vi "Input impedance.vi"() -> ()   [LabVIEW 2017]
panel:
  out "ph1-ph2":dbl
  out "A2":dbl
  out "A1":dbl
  out "ph1-ph2 graph":cluster{"Y":dbl[], "Y":dbl[]}[](graph)
  out "A2 graph":cluster{"Y":dbl[], "Y":dbl[]}[](graph)
  out "A1 graph":cluster{"Y":dbl[], "Y":dbl[]}[](graph)
  out "Im Z 2":dbl=nan
  out "Re Z 2":dbl=nan
  out "Im (Z)":cluster{"Y":dbl[], "Y":dbl[]}[](graph)
  out "Re (Z)":cluster{"Y":dbl[], "Y":dbl[]}[](graph)
  out "Arg (Z)":cluster{"Y":dbl[], "Y":dbl[]}[](graph)
  out "Abs (Z)":cluster{"Y":dbl[], "Y":dbl[]}[](graph)
  out "Abs Z 2":dbl=nan
  out "Arg Z 2":dbl=nan
  in  "Resistance (Ohm)":dbl=162.0
  in  "Commentary":string
  in  "horiz range factor":dbl=0.3
  in  "vert range factor":dbl=1.2
  out "frequency":dbl=20010000.0
  out "datafile":refnum<file>
  in  "Min f":dbl=10000.0
  in  "Channel 2 preset commands":string=":channel2:bwlimit 0\n:channel2:coupling AC\n:channel2:display 1\n:channel2:invert 0\n:channel2:offset 0"
  in  "Channel 1 preset commands":string=":channel1:bwlimit 0\n:channel1:coupling AC\n:channel1:display 1\n:channel1:invert 0\n:channel1:offset 0\n"
  in  "Ampl":dbl=9.0
  in  "Source preset commands":string=":WGEN:OUTPut 1\n:WGEN:VOLTage:OFFSet 1e-6\n:WGEN:OUTPut:LOAD FIFTy\n:wgen:function sinusoid\n:WGEN:OUTPut:POLarity 0\n"
  in  "Delta f":dbl=10000.0
  in  "Max f":dbl=20000000.0
  in  "Timeout Value (ms)":u32=5000
  in  "VISA resource name":refnum<visa-resource-name>="USB0::0x2A8D::0x1797::CN58056487::INSTR"
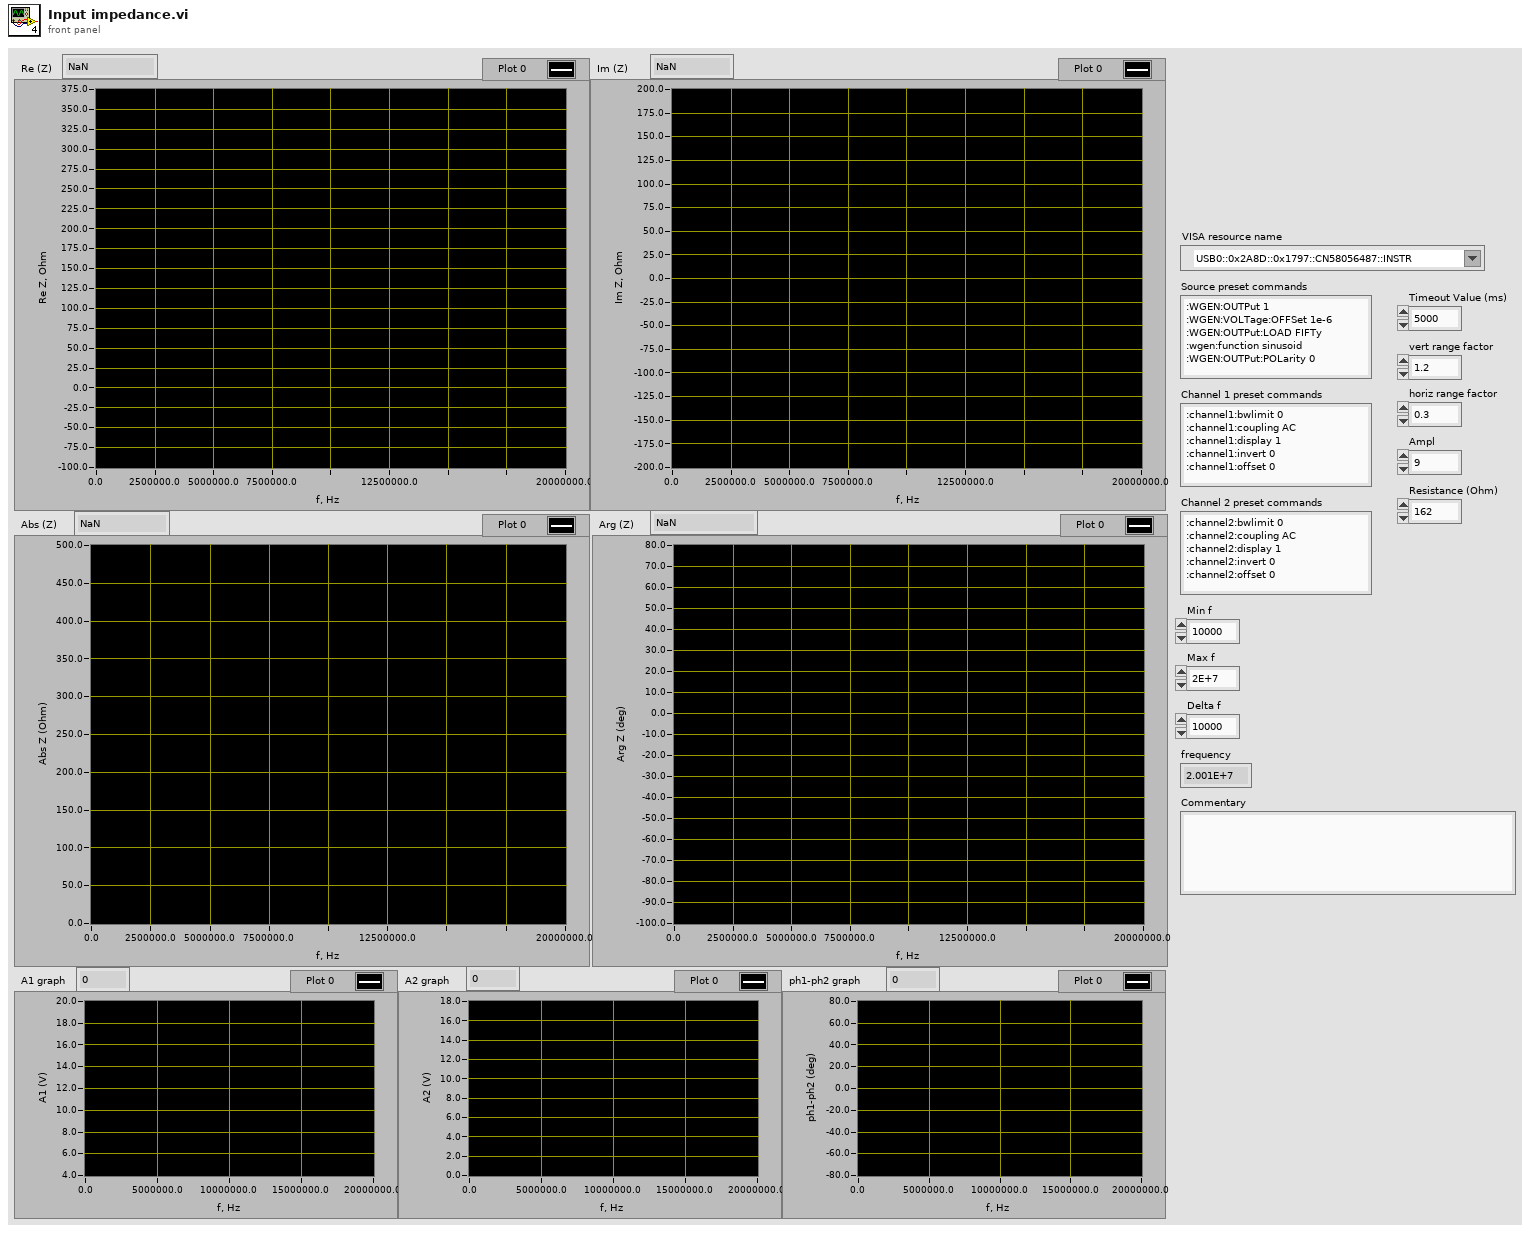
[diagram p1: front panel]
types:
  T1 = enum16{"open", "replace", "create", "open or create", "replace or create", "replace or create with confirmation"}
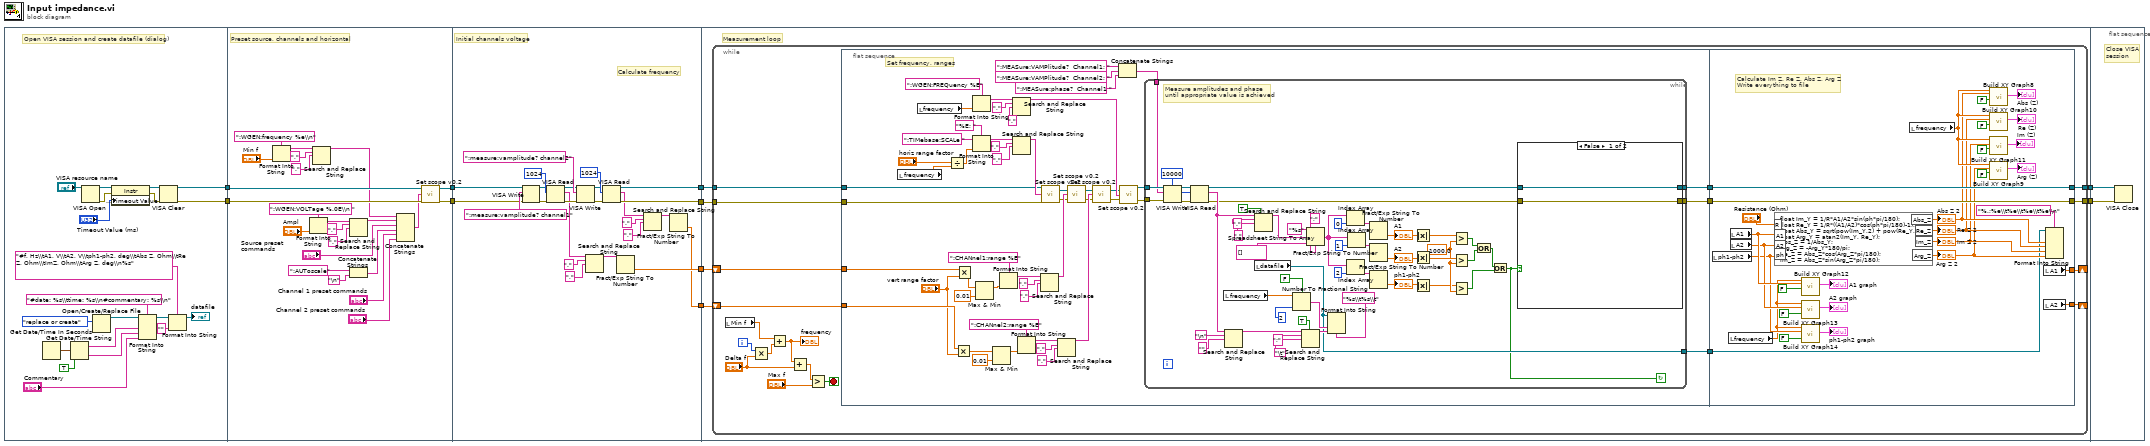
[diagram p0: block diagram]
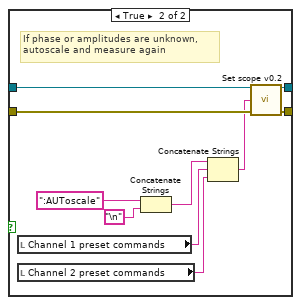
[diagram p2: hidden frame]
diagram:
  n1 = flat-sequence {
    tunnel: [w23] -> w10
    tunnel: [w24] -> w9
    tunnel: [w53] -> w8
    tunnel: [w52] -> w7
    tunnel: w9 -> [w50]
    tunnel: w10 -> [w51]
    tunnel: w8 -> [w67]
    tunnel: w7 -> [w66]
    tunnel: [w59] -> w6
    tunnel: [w54] -> w5
    tunnel: [w65] -> w4
    tunnel: [w64] -> w3
    tunnel: w6 -> [w83]
    tunnel: w5 -> [w82]
    tunnel: w4 -> [w81]
    tunnel: w3 -> [w80]
    tunnel: [w79] -> w2
    tunnel: [w78] -> w1
    tunnel: w2 -> [w247]
    tunnel: w1 -> [w246]
    frame #0 {
      # "Open VISA session and create datafile (dialog)"
      n2 = Get Date/Time In Seconds() -> (seconds since 1Jan1904=w20:timestamp)
      n3 = Get Date/Time String(seconds (now)=w20, want seconds? (F)=TRUE) -> (date string=w17:string, time string=w16:string)  [unwired: 1 in]
      n4 = VISA Open(VISA resource name="VISA resource name") -> (VISA resource name=w28:refnum<visa-resource-name>, error out=w29:errorcluster)  [unwired: 4 in]
      n5 = Open/Create/Replace File(operation (0:open)=T1."replace or create") -> (refnum out=w21:refnum<file>)  [unwired: 5 in, 2 out]
      n6 = property class="Instr"(reference=w28, error in=w29, "General Settings:Timeout Value"="Timeout Value (ms)") -> (reference out=w26:refnum<visa-resource-name>, error out=w25:errorcluster)
      n7 = Format Into String(format string="#date: %s\\ttime: %s\\n#commentary: %s\\n", initial string=w21, w17, w16, "Commentary") -> (resulting string=w13:refnum<file>)  [unwired: 1 in, 1 out]
      n8 = VISA Clear(VISA resource name=w26, error in (no error)=w25) -> (VISA resource name out=w23:refnum<visa-resource-name>, error out=w24:errorcluster)
      n9 = Format Into String(format string="#f, Hz\\tA1, V\\tA2, V\\tph1-ph2, deg\\tAbs Z, Ohm\\tRe Z, Ohm\\tImZ, Ohm\\tArg Z, deg\\n%s", initial string=w13, "" ("input 1")) -> (resulting string=→"datafile":refnum<file>)  [unwired: 1 in, 1 out]
    }
    frame #1 {
      # "Preset source, channels and horizontal"
      n10 = Format Into String(format string=":WGEN:frequency %e\\n", "Min f") -> (resulting string=w39:string)  [unwired: 2 in, 1 out]
      n11 = Format Into String(format string=":WGEN:VOLTage %.0E\\n ", "Ampl") -> (resulting string=w45:string)  [unwired: 2 in, 1 out]
      n12 = Search and Replace String(input string=w39, search string="," ("replace string (\"\")"), replace string="." ("replace string (\"\")")) -> (result string=w36:string)  [unwired: 5 in, 3 out]
      n13 = Search and Replace String(input string=w45, search string="," ("replace string (\"\")"), replace string="." ("replace string (\"\")")) -> (result string=w43:string)  [unwired: 5 in, 3 out]
      n14 = Concatenate Strings(":AUToscale" ("write buffer"), "\n") -> (w33:string)
      n15 = Concatenate Strings(w36, w43, "Source preset commands", w33, "Channel 1 preset commands", "Channel 2 preset commands") -> (w44:string)
      n16 = call "Set scope v0.2.vi"("error in (no error)"=w50, "input commands"=w44, "VISA resource name in"=w51) -> ("error out"=w52:errorcluster, "VISA resource name out"=w53:refnum<visa-resource-name>)
    }
    frame #2 {
      # "Calculate frequency"
      # "Initial channels voltage"
      n17 = VISA Write(VISA resource name=w67, write buffer=":measure:vamplitude? channel1", error in (no error)=w66) -> (VISA resource name out=w71:refnum<visa-resource-name>, error out=w70:errorcluster)  [unwired: 1 out]
      n18 = VISA Read(VISA resource name=w71, byte count=u32 1024, error in (no error)=w70) -> (VISA resource name out=w72:refnum<visa-resource-name>, read buffer=w61:string, error out=w73:errorcluster)  [unwired: 1 out]
      n19 = VISA Write(VISA resource name=w72, write buffer=":measure:vamplitude? channel2", error in (no error)=w73) -> (VISA resource name out=w69:refnum<visa-resource-name>, error out=w68:errorcluster)  [unwired: 1 out]
      n20 = Search and Replace String(input string=w61, search string="." ("replace string (\"\")"), replace string="," ("replace string (\"\")")) -> (result string=w60:string)  [unwired: 5 in, 3 out]
      n21 = VISA Read(VISA resource name=w69, byte count=u32 1024, error in (no error)=w68) -> (VISA resource name out=w65:refnum<visa-resource-name>, read buffer=w55:string, error out=w64:errorcluster)  [unwired: 1 out]
      n22 = Fract/Exp String To Number(string=w60) -> (number=w59:dbl)  [unwired: 3 in, 1 out]
      n23 = Search and Replace String(input string=w55, search string="." ("replace string (\"\")"), replace string="," ("replace string (\"\")")) -> (result string=w56:string)  [unwired: 5 in, 3 out]
      n24 = Fract/Exp String To Number(string=w56) -> (number=w54:dbl)  [unwired: 3 in, 1 out]
    }
    frame #3 {
      # "Measurement loop"
      n25 = while {
        shift-right: [w92] -> _
        shift-left: w83 -> [w102]
        shift-right: [w93] -> _
        shift-left: w82 -> [w101]
        tunnel: w81 -> [w100]
        tunnel: w80 -> [w99]
        tunnel: [w98] -> w79
        tunnel: [w97] -> w78
        i -> [w87]
        stop <- w89 stop-if-true
        n26 = local read "Min f"() -> (w91:dbl)
        n27 = Multiply(x=w87, y="Delta f") -> (x*y=w90:dbl)
        n28 = Add(x=w91, y=w90) -> (x+y=w88:dbl)
        "frequency" <- w88
        n29 = Add(x=w88, y="Delta f") -> (x+y=w85:dbl)
        n30 = Greater?(x=w85, y="Max f") -> (0:w89:bool)
        n31 = flat-sequence {
          tunnel: [w105] -> w95
          tunnel: [w103] -> w96
          tunnel: [w104] -> w94
          tunnel: w99 -> [w122]
          tunnel: w100 -> [w123]
          tunnel: w101 -> [w120]
          tunnel: w102 -> [w121]
          tunnel: [w244] -> w97
          tunnel: [w245] -> w98
          tunnel: w95 -> [w245]
          tunnel: w96 -> [w222]
          tunnel: w94 -> [w244]
          tunnel: [w217] -> w93
          tunnel: [w216] -> w92
          frame #0 {
            # "Set frequency, ranges"
            n32 = local read "frequency"() -> (w128:dbl)
            n33 = local read "frequency"() -> (w129:dbl)
            n34 = Divide(x="horiz range factor", y=w128) -> (x/y=w148:dbl)
            n35 = Multiply(x=w120, y="vert range factor") -> (x*y=w133:dbl)
            n36 = Multiply(x=w121, y="vert range factor") -> (x*y=w139:dbl)
            n37 = Format Into String(format string="%E; ", initial string=":TIMebase:SCALe " ("write buffer"), w148) -> (resulting string=w149:string)  [unwired: 1 in, 1 out]
            n38 = Format Into String(format string=":WGEN:FREQuency %E", w129) -> (resulting string=w152:string)  [unwired: 2 in, 1 out]
            n39 = Max & Min(x=w139, y=0.01) -> (max(x,y)=w137:dbl)  [unwired: 1 out]
            n40 = Max & Min(x=w133, y=0.01) -> (max(x,y)=w131:dbl)  [unwired: 1 out]
            n41 = Format Into String(format string=":CHANnel1:range %E", w137) -> (resulting string=w143:string)  [unwired: 2 in, 1 out]
            n42 = Search and Replace String(input string=w152, search string="," ("replace string (\"\")"), replace string="." ("replace string (\"\")")) -> (result string=w115:string)  [unwired: 5 in, 3 out]
            n43 = Search and Replace String(input string=w149, search string="," ("replace string (\"\")"), replace string="." ("replace string (\"\")")) -> (result string=w127:string)  [unwired: 5 in, 3 out]
            n44 = Format Into String(format string=":CHANnel2:range %E", w131) -> (resulting string=w136:string)  [unwired: 2 in, 1 out]
            n45 = Search and Replace String(input string=w143, search string="," ("replace string (\"\")"), replace string="." ("replace string (\"\")")) -> (result string=w126:string)  [unwired: 5 in, 3 out]
            n46 = call "Set scope v0.2.vi"("error in (no error)"=w122, "input commands"=w127, "VISA resource name in"=w123) -> ("error out"=w125:errorcluster, "VISA resource name out"=w124:refnum<visa-resource-name>)
            n47 = Search and Replace String(input string=w136, search string="," ("replace string (\"\")"), replace string="." ("replace string (\"\")")) -> (result string=w118:string)  [unwired: 5 in, 3 out]
            n48 = call "Set scope v0.2.vi"("error in (no error)"=w125, "input commands"=w126, "VISA resource name in"=w124) -> ("error out"=w117:errorcluster, "VISA resource name out"=w116:refnum<visa-resource-name>)
            n49 = call "Set scope v0.2.vi"("error in (no error)"=w117, "input commands"=w118, "VISA resource name in"=w116) -> ("error out"=w113:errorcluster, "VISA resource name out"=w114:refnum<visa-resource-name>)
            n50 = Concatenate Strings(":MEASure:VAMPlitude?  Channel1; " ("write buffer"), ":MEASure:VAMPlitude?  Channel2; " ("write buffer"), ":MEASure:phase?  Channel1 " ("write buffer")) -> (w106:string)
            n51 = call "Set scope v0.2.vi"("error in (no error)"=w113, "input commands"=w115, "VISA resource name in"=w114) -> ("error out"=w110:errorcluster, "VISA resource name out"=w111:refnum<visa-resource-name>)
            n52 = while {
              tunnel: w111 -> [w165]
              tunnel: w110 -> [w164]
              tunnel: w106 -> [w163]
              tunnel: [w162] -> w105
              tunnel: [w161] -> w104
              tunnel: [w160] -> w103
              stop <- w154 continue-if-true
              w158 = 1000.0 ("y")
              # "Measure amplitudes and phase\nuntil appropriate value is achieved"
              n53 = VISA Write(VISA resource name=w165, write buffer=w163, error in (no error)=w164) -> (VISA resource name out=w203:refnum<visa-resource-name>, error out=w202:errorcluster)  [unwired: 1 out]
              n54 = VISA Read(VISA resource name=w203, byte count=u32 10000, error in (no error)=w202) -> (VISA resource name out=w187:refnum<visa-resource-name>, read buffer=w193:string, error out=w186:errorcluster)  [unwired: 1 out]
              n55 = local read "frequency"() -> (w194:dbl)
              n56 = Search and Replace String(input string=w193, search string="\n", replace string="" ("replace string (\"\")")) -> (result string=w192:string)  [unwired: 5 in, 3 out]
              n57 = Search and Replace String(replace all?=TRUE ("replace all? (F)"), input string=w193, search string="." ("replace string (\"\")"), replace string="," ("replace string (\"\")")) -> (result string=w201:string)  [unwired: 4 in, 3 out]
              n58 = local read "datafile"() -> (w160:refnum<file>)
              n59 = Number To Fractional String(use system decimal point (T)=FALSE, number=w194, precision (6)=i16 2) -> (F-format string=w197:string)  [unwired: 1 in]
              n60 = Search and Replace String(replace all?=TRUE ("replace all? (F)"), input string=w192, search string=";", replace string="\t") -> (result string=w198:string)  [unwired: 4 in, 3 out]
              n61 = Spreadsheet String To Array(delimiter (Tab)=";", format string="%s", spreadsheet string=w201, array type (2D Dbl)=string[] [] ("initialized array")) -> (array=w196:string[])
              n62 = Format Into String(format string="%s\\t%s\\t", initial string=w160, w197, w198) -> ()  [unwired: 1 in, 2 out]
              n63 = Index Array(array=w196, index=0) -> (element=w200:string)
              n64 = Index Array(array=w196, index=2) -> (element=w195:string)
              n65 = Index Array(array=w196, index=1) -> (element=w199:string)
              n66 = Fract/Exp String To Number(string=w200) -> (number=w191:dbl)  [unwired: 3 in, 1 out]
              "A1" <- w191
              n67 = Fract/Exp String To Number(string=w199) -> (number=w190:dbl)  [unwired: 3 in, 1 out]
              "A2" <- w190
              n68 = Fract/Exp String To Number(string=w195) -> (number=w159:dbl)  [unwired: 3 in, 1 out]
              "ph1-ph2" <- w159
              n69 = Absolute Value(x=w191) -> (abs(x)=w189:dbl)
              n70 = Absolute Value(x=w190) -> (abs(x)=w188:dbl)
              n71 = Absolute Value(x=w159) -> (abs(x)=w157:dbl)
              n72 = Greater?(x=w189, y=w158) -> (0:w185:bool)
              n73 = Greater?(x=w188, y=w158) -> (0:w184:bool)
              n74 = Greater?(x=w157, y=w158) -> (0:w156:bool)
              n75 = Or(x=w185, y=w184) -> (x .or. y?=w155:bool)
              n76 = Or(x=w155, y=w156) -> (x .or. y?=w154:bool)
              n77 = case shown="False" w154 {
                tunnel: w187 -> [w205 w213]
                tunnel: w186 -> [w204 w212]
                tunnel: [w204 w211] -> w161
                tunnel: [w205 w210] -> w162
                frame False {
                }
                frame True {
                  # "If phase or amplitudes are unknown, \nautoscale and measure again"
                  n78 = local read "Channel 1 preset commands"() -> (w208:string)
                  n79 = local read "Channel 2 preset commands"() -> (w207:string)
                  n80 = Concatenate Strings(":AUToscale" ("write buffer"), "\n") -> (w209:string)
                  n81 = Concatenate Strings(w209, w208, w207) -> (w206:string)
                  n82 = call "Set scope v0.2.vi"("error in (no error)"=w212, "input commands"=w206, "VISA resource name in"=w213) -> ("error out"=w211:errorcluster, "VISA resource name out"=w210:refnum<visa-resource-name>)
                }
              }
            }
          }
          frame #1 {
            # "Calculate Im Z, Re Z, Abs Z, Arg Z\nWrite everything to file"
            n83 = local read "ph1-ph2"() -> (w219:dbl)
            n84 = local read "frequency"() -> (w218:dbl)
            n85 = local read "A1"() -> (w221:dbl)
            n86 = local read "A2"() -> (w220:dbl)
            n87 = formula code="float Im_Y = 1/R*A1/A2*sin(ph*pi/180);\nfloat Re_Y = 1/R*((A1/A2)*cos(ph*pi/180)-1);\nfloat Abs_Y = sqrt(pow(Im_Y,2) + pow(Re_Y,2));\nfloat Arg_Y = atan2(Im_Y, Re_Y);\nAbs_Z = 1/Abs_Y;\nArg_Z = -Arg_Y*180/pi;\nRe_Z = Abs_Z*cos(Arg_Z*pi/180);\nIm_Z = Abs_Z*sin(Arg_Z*pi/180);"("R"="Resistance (Ohm)", "A1"=w221, "A2"=w220, "ph"=w219) -> ("Im_Z"=w224:dbl, "Arg_Z"=w223:dbl, "Re_Z"=w225:dbl, "Abs_Z"=w226:dbl)
            "Arg Z 2" <- w223
            "Abs Z 2" <- w226
            "Re Z 2" <- w225
            "Im Z 2" <- w224
            n88 = call "Build XY Graph12"("Reset"=FALSE, "Y Input"=w221, "X Input"=w218) -> ("XY Graph"=→"A1 graph":cluster{"X":dbl[], "Y":dbl[]}[])  [unwired: 7 in, 1 out]
            n89 = call "Build XY Graph13"("Reset"=FALSE, "Y Input"=w220, "X Input"=w218) -> ("XY Graph"=→"A2 graph":cluster{"X":dbl[], "Y":dbl[]}[])  [unwired: 7 in, 1 out]
            n90 = call "Build XY Graph14"("Reset"=FALSE, "Y Input"=w219, "X Input"=w218) -> ("XY Graph"=→"ph1-ph2 graph":cluster{"X":dbl[], "Y":dbl[]}[])  [unwired: 7 in, 1 out]
            n91 = local read "frequency"() -> (w227:dbl)
            n92 = call "Build XY Graph8"("Reset"=FALSE, "Y Input"=w226, "X Input"=w227) -> ("XY Graph"=→"Abs (Z)":cluster{"X":dbl[], "Y":dbl[]}[])  [unwired: 7 in, 1 out]
            n93 = call "Build XY Graph10"("Reset"=FALSE, "Y Input"=w225, "X Input"=w227) -> ("XY Graph"=→"Re (Z)":cluster{"X":dbl[], "Y":dbl[]}[])  [unwired: 7 in, 1 out]
            n94 = call "Build XY Graph11"("Reset"=FALSE, "Y Input"=w224, "X Input"=w227) -> ("XY Graph"=→"Im (Z)":cluster{"X":dbl[], "Y":dbl[]}[])  [unwired: 7 in, 1 out]
            n95 = call "Build XY Graph9"("Reset"=FALSE, "Y Input"=w223, "X Input"=w227) -> ("XY Graph"=→"Arg (Z)":cluster{"X":dbl[], "Y":dbl[]}[])  [unwired: 7 in, 1 out]
            n96 = local read "A1"() -> (w216:dbl)
            n97 = local read "A2"() -> (w217:dbl)
            n98 = Format Into String(format string="%.;%e\\t%e\\t%e\\t%e\\n", initial string=w222, w226, w225, w224, w223) -> ()  [unwired: 1 in, 2 out]
          }
        }
      }
    }
    frame #4 {
      # "Close VISA\nsession"
      n99 = VISA Close(VISA resource name=w247, error in (no error)=w246) -> ()  [unwired: 1 out]
    }
  }
